vi "Release.vi"(8 "Error In":errorcluster, 11 "Int In":refnum<class "Integer.lvclass">) -> (0 "Error Out":errorcluster)   [LabVIEW 2016, in "Integer.lvclass"]
uses:
  Integer.lvclass
  Tree Data/Tree Data.lvclass
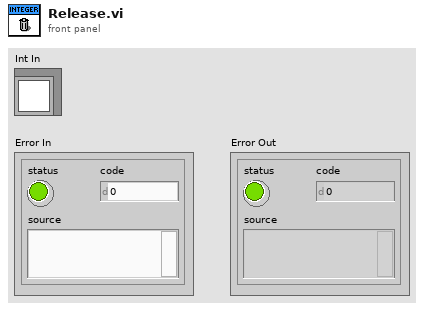
[diagram p1: front panel]
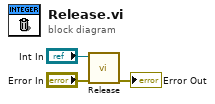
[diagram p0: block diagram]
diagram:
  n1 = call-parent "Release.vi"("Error In"="Error In", "Tree Data In"="Int In") -> ("Error Out"=→"Error Out":errorcluster)  [unwired: 9 in]
